vi "Read Local Files.vi"(6 "Error Message in":string, 8 "Error In":errorcluster, 11 "Full App Name":string="PC Interface.exe") -> (0 "Error Out":errorcluster, 2 "Local Version Array":i32[](array[numeric]), 4 "Error Message out":string)   [LabVIEW 2019]
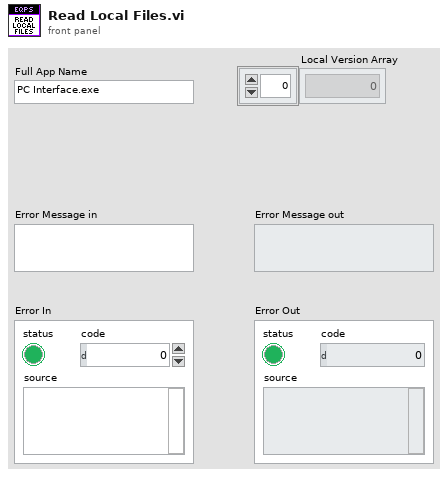
[diagram p1: front panel]
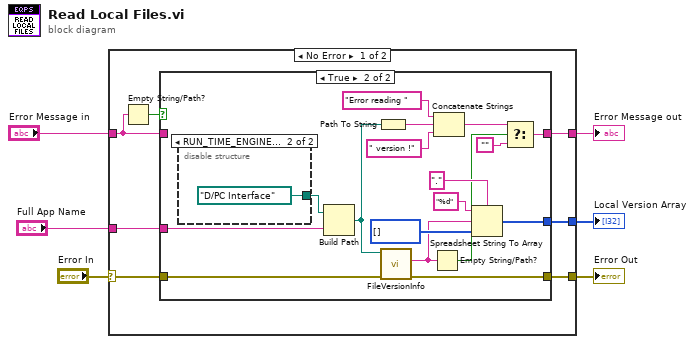
[diagram p0: block diagram]
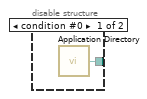
[diagram p3: hidden frame]
diagram:
  n1 = case shown="No Error" "Error In" {
    selector: "Error In" -> [w9 w36]
    tunnel: [w10 w36] -> w5
    tunnel: [w12 w35] -> w4
    tunnel: "Error Message in" -> [w11 w35]
    tunnel: [w8 _] -> w2
    tunnel: "Full App Name" -> [w7 _]
    frame No Error {
      n2 = Empty String/Path?(string/path=w11) -> (empty?=w13:bool)
      n3 = case shown="True" w13 {
        tunnel: [w15 w18] -> w12
        tunnel: w11 -> [w15 _]
        tunnel: [w14 w26] -> w10
        tunnel: w9 -> [w14 w31]
        tunnel: [_ w17] -> w8
        tunnel: w7 -> [_ w16]
        frame False {
        }
        frame True {
          n4 = disable-structure shown="RUN_TIME_ENGINE==False" {
            disable-tunnel: [w33 path "D:/PC Interface"] -> w32
            frame condition #0 {
              n5 = call <vilib>:"Application Directory.vi"() -> ("Application Directory"=w33:path)
            }
            frame condition #1 (active) {
            }
          }
          n6 = Build Path(base path=w32, name or relative path=w16) -> (appended path=w23:path)
          n7 = Path To String(path=w23) -> (string=w22:string)
          n8 = call <vilib>:"FileVersionInfo.vi"("error in (no error)"=w31, "Application Path in"=w23) -> ("error out"=w26:errorcluster, "File Version Info"=w27:string)  [unwired: 6 in, 2 out]
          n9 = Empty String/Path?(string/path=w27) -> (empty?=w21:bool)
          n10 = Concatenate Strings("Error reading ", w22, " version !") -> (w20:string)
          n11 = Spreadsheet String To Array(delimiter (Tab)=".", format string="%d", spreadsheet string=w27, array type (2D Dbl)=i32[] []) -> (array=w17:i32[])
          n12 = Select(t=w20, s=w21, f="") -> (s? t:f=w18:string)
        }
      }
    }
    frame Error {
    }
  }
  "Error Out" <- w5
  "Error Message out" <- w4
  "Local Version Array" <- w2
